vi "ReadUnixPathFromFile.vi"(10 "relative":bool=TRUE, 11 "path":string) -> (3 "path":path)   [LabVIEW 2009, in "NavScreen.lvlib"]
uses:
  NavScreen.lvlib
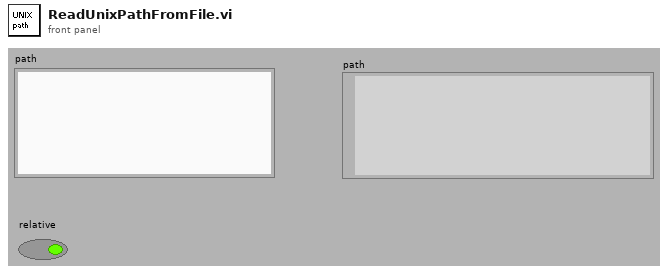
[diagram p1: front panel]
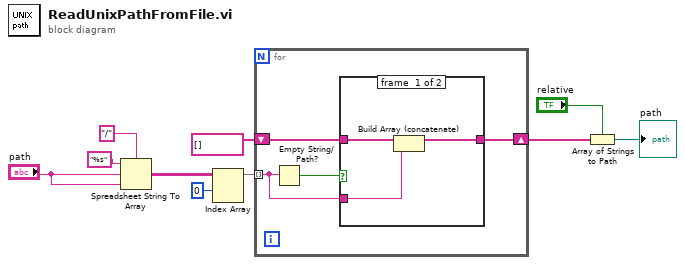
[diagram p0: block diagram]
diagram:
  n1 = Spreadsheet String To Array(delimiter (Tab)="/", format string="%s", spreadsheet string="path", array type (2D Dbl)="path") -> (array=w6:string[][])
  n2 = Index Array(array=w6, index (row)=0) -> (element=w4:string[])  [unwired: 1 in]
  n3 = for {
    tunnel: w4 -> [w11] mode=indexing
    shift-right: [w12] -> w3
    shift-left: string[] [] -> [w13]
    n4 = Empty String/Path?(string/path=w11) -> (empty?=w14:bool)
    n5 = case shown="False" w14 {
      tunnel: w13 -> [w17 w18]
      tunnel: [w15 w18] -> w12
      tunnel: w11 -> [w16 _]
      frame #0 {
        n6 = Build Array (concatenate)(w17, w16) -> (w15:string[])
      }
      frame #1 {
      }
    }
  }
  n7 = Array of Strings to Path(0:w3, 1:"relative") -> (2:→"path":path)
